vi "MTDC_Prototype.vi"() -> ()   [LabVIEW 2025]
uses:
  STM-Auto-Project/QMH CTLS/Scan_Params (QMH).ctl
  <instrlib>/SMS LabVIEW Drivers/Source Code/Public/PSU Status.ctl
  <instrlib>/SMS LabVIEW Drivers/Source Code/Cryogenic Ltd SMSXXX.lvlib
  Downloads/OneDrive_2025-09-03/Instrument Controls/Temp Cntrl.ctl
  STM-Auto-Project/QMH CTLS/Sweeper.ctl
  Magnetic Drift Correction/XY_Coords(Final).ctl
panel:
  out "Polled Temps (K)":dbl[](array[numeric])
  in  "Serial Configuration":T1={"Baud Rate"=57600, "Parity"=1, "Data Bits"=7, "Stop Bits"=10, "Flow Control"=0}
  out "Translation (m)":T2
  out "Final coordinates (m)":cluster{"Xc":sgl, "Yc":sgl} {"Yc" format="%.4p"; "Xc" format="%.4p"}
  out "Initial coordinates (m)":cluster{"Xc":sgl, "Yc":sgl} {"Yc" format="%.4p"; "Xc" format="%.4p"}
  in  "Field and Temp Range":T3={"VISA (Magnet)"="COM4", "Fields(T)"=[], "Temps(K)"=[], "VISA (Temp) "="COM1", "Port number (3364)"=3364}
  in  "Lead- Mode Ramp Rate (A/s)":dbl=0.02
  out "Errors":errorcluster[](array[cluster])
  out "Output (T)":dbl
  in  "P-Mode Ramp Rate (A/s)":dbl
  out "MID Setpoint (T)":dbl
  out "Current Index":i32
  in  "stop":bool
  in  "Start":bool
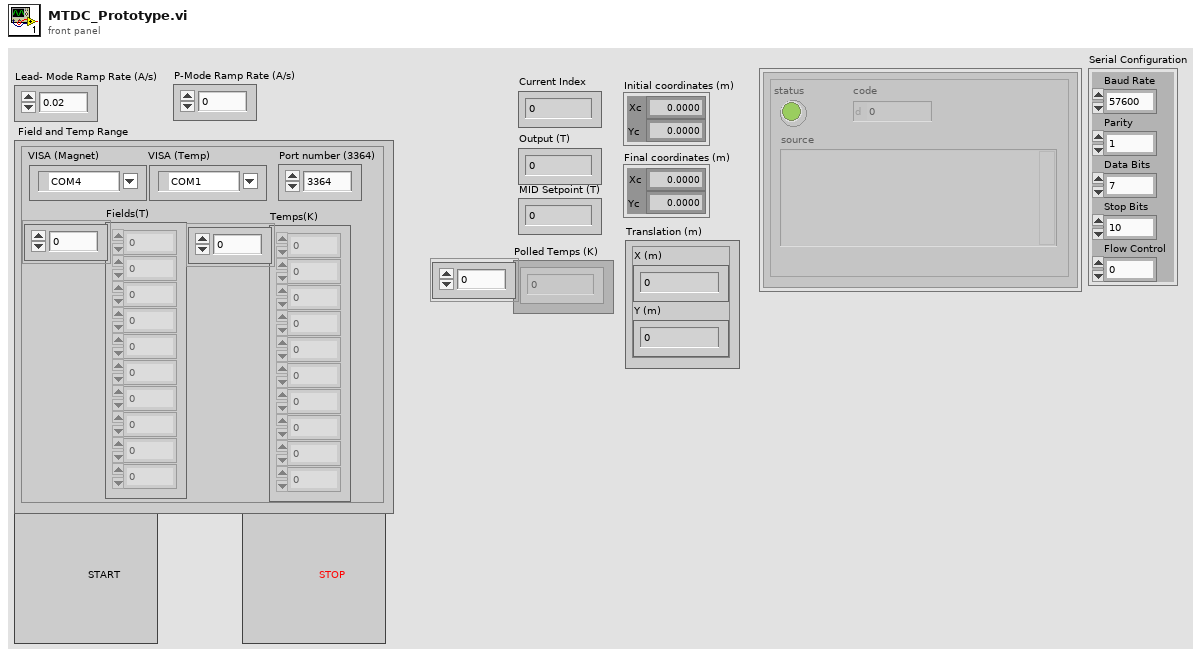
[diagram p1: front panel]
types:
  T1 = cluster{"Baud Rate":u32, "Parity":u16, "Data Bits":u16, "Stop Bits":u16, "Flow Control":u16}
  T2 = typedef "XY_Coords(Final).ctl" = cluster{"X (m)":dbl, "Y (m)":dbl}
  T3 = cluster{"VISA (Magnet)":refnum<visa-resource-name>, "Fields(T)":dbl[], "Temps(K)":dbl[], "VISA (Temp) ":refnum<visa-resource-name>, "Port number (3364)":u32}
  T4 = enum16{"NO CHANGE", "SET TEMP & FIELD", "SWEEP IDLE", "NEXT TEMP & FIELD", "SWEEP DONE"}
  T5 = enum16{"1. BIAS", "2. INIT_SCAN", "3. SCAN_IDLE", "4. INTER_SCAN", "5. NEW_COORDS_&_FRAME", "6. FINAL_SCAN", "7. POLL BIAS ", "8. STOP"}
  T6 = typedef "Sweeper.ctl" = cluster{"Temps(K)":dbl[], "Fields(T)":dbl[], "Sweep States":enum16{"NO CHANGE", "SET TEMP & FIELD", "SWEEP IDLE", "NEXT TEMP & FIELD", "SWEEP DONE"}}
  T7 = enum16{"1. INIT TEMP", "2. TC ON", "3. POLL_TEMPS", "4. TEMP_STAB", "5. TC IDLE", "6. APPLY NEXT TEMP", "7. TC OFF (Reset)"}
  T8 = typedef "Temp Cntrl.ctl" = cluster{"Range (0:Off)":u16, "Manual Output (0.00 %)":dbl, "Rate (D) (0.0 %)":dbl, "Reset (I) (20.0)":dbl, "Gain (P) (50.0)":dbl, "Power Up Enable (F: Disable)":bool, "Max User Current (2.000)":dbl, "Heater Resistance (1:25 Ohms)":u16, "Max Current (0:User Specified)":u16, "Heater Out Display (1:Current)":u16, "Mode (0:Off)":u16, "Input (0:None)":u16, "Target Temp (K)":dbl, "Serial Configuration":cluster{"Baud Rate":u32, "Parity":u16, "Data Bits":u16, "Stop Bits":u16, "Flow Control":u16}, "VISA resource name":refnum<visa-resource-name>, "Configure Control Parameters (0: Configure)":u16, "Enable Setpoint (F:Disable)":bool, "Input (0:A)":u16, "Data Source (0:Kelvin)":u16, "Output's Control Loop (1:1)":u16, "STND DEV Threshold ":dbl, "Mean Tolerance ":dbl, "Current State":enum16{"1. INIT TEMP", "2. TC ON", "3. POLL_TEMPS", "4. TEMP_STAB", "5. TC IDLE", "6. APPLY NEXT TEMP", "7. TC OFF (Reset)"}}
  T9 = enum16{"1. INIT MAG", "2. MAG ON", "3. MAG_STAB", "4. MAG IDLE", "5. PREP NEXT FIELD", "6. APPLY NEXT FIELD", "7. PREP OFF", "8. MAG OFF (Reset)"}
  T10 = typedef "PSU Status.ctl" = cluster{"Ramp Target":enum16{"ZERO", "MID", "MAX"}, "Pause":bool, "Switch Heater":bool, "Persistent Field":dbl, "Persistent Current":dbl, "Tesla":bool, "Output (T)":dbl, "Output (A)":dbl, "X Trip":enum16{"DISABLED", "ENABLED", "ACTIVE"}, "Ramp Rate (A/s)":dbl, "V Limit (V)":dbl, "Heater Voltage":dbl, "MAX Setpoint (A)":dbl, "MAX Setpoint (T)":dbl, "MID Setpoint (A)":dbl, "MID Setpoint (T)":dbl, "Lock":bool, "Field Constant":dbl, "Remote":bool, "Direction":enum16{"POSITIVE", "NEGATIVE", "OPEN", "UNIPOLAR"}, "Helium Level":u16, "Quench !":bool, "Voltage":dbl, "V Limit !":bool, "Ramping":bool, "At Target":bool, "Trip Field":dbl, "Trip Current":dbl, "Current State":enum16{"1. INIT MAG", "2. MAG ON", "3. MAG_STAB", "4. MAG IDLE", "5. PREP NEXT FIELD", "6. APPLY NEXT FIELD", "7. PREP OFF", "8. MAG OFF (Reset)"}, "MAG Reference":refnum<visa-resource-name>}
  T11 = typedef "Scan_Params (QMH).ctl" = cluster{"Setpoint (I)":dbl[], "Bias (V)":dbl[], "Number of scans":u8, "Port number (3364)":u32, "Avoid zero threshold (V)":dbl, "Current State":enum16{"1. BIAS", "2. INIT_SCAN", "3. SCAN_IDLE", "4. INTER_SCAN", "5. NEW_COORDS_&_FRAME", "6. FINAL_SCAN", "7. POLL BIAS ", "8. STOP"}}
  T12 = enum16{"RAMP TO ZERO", "RAMP TO MID", "RAMP TO MAX"}
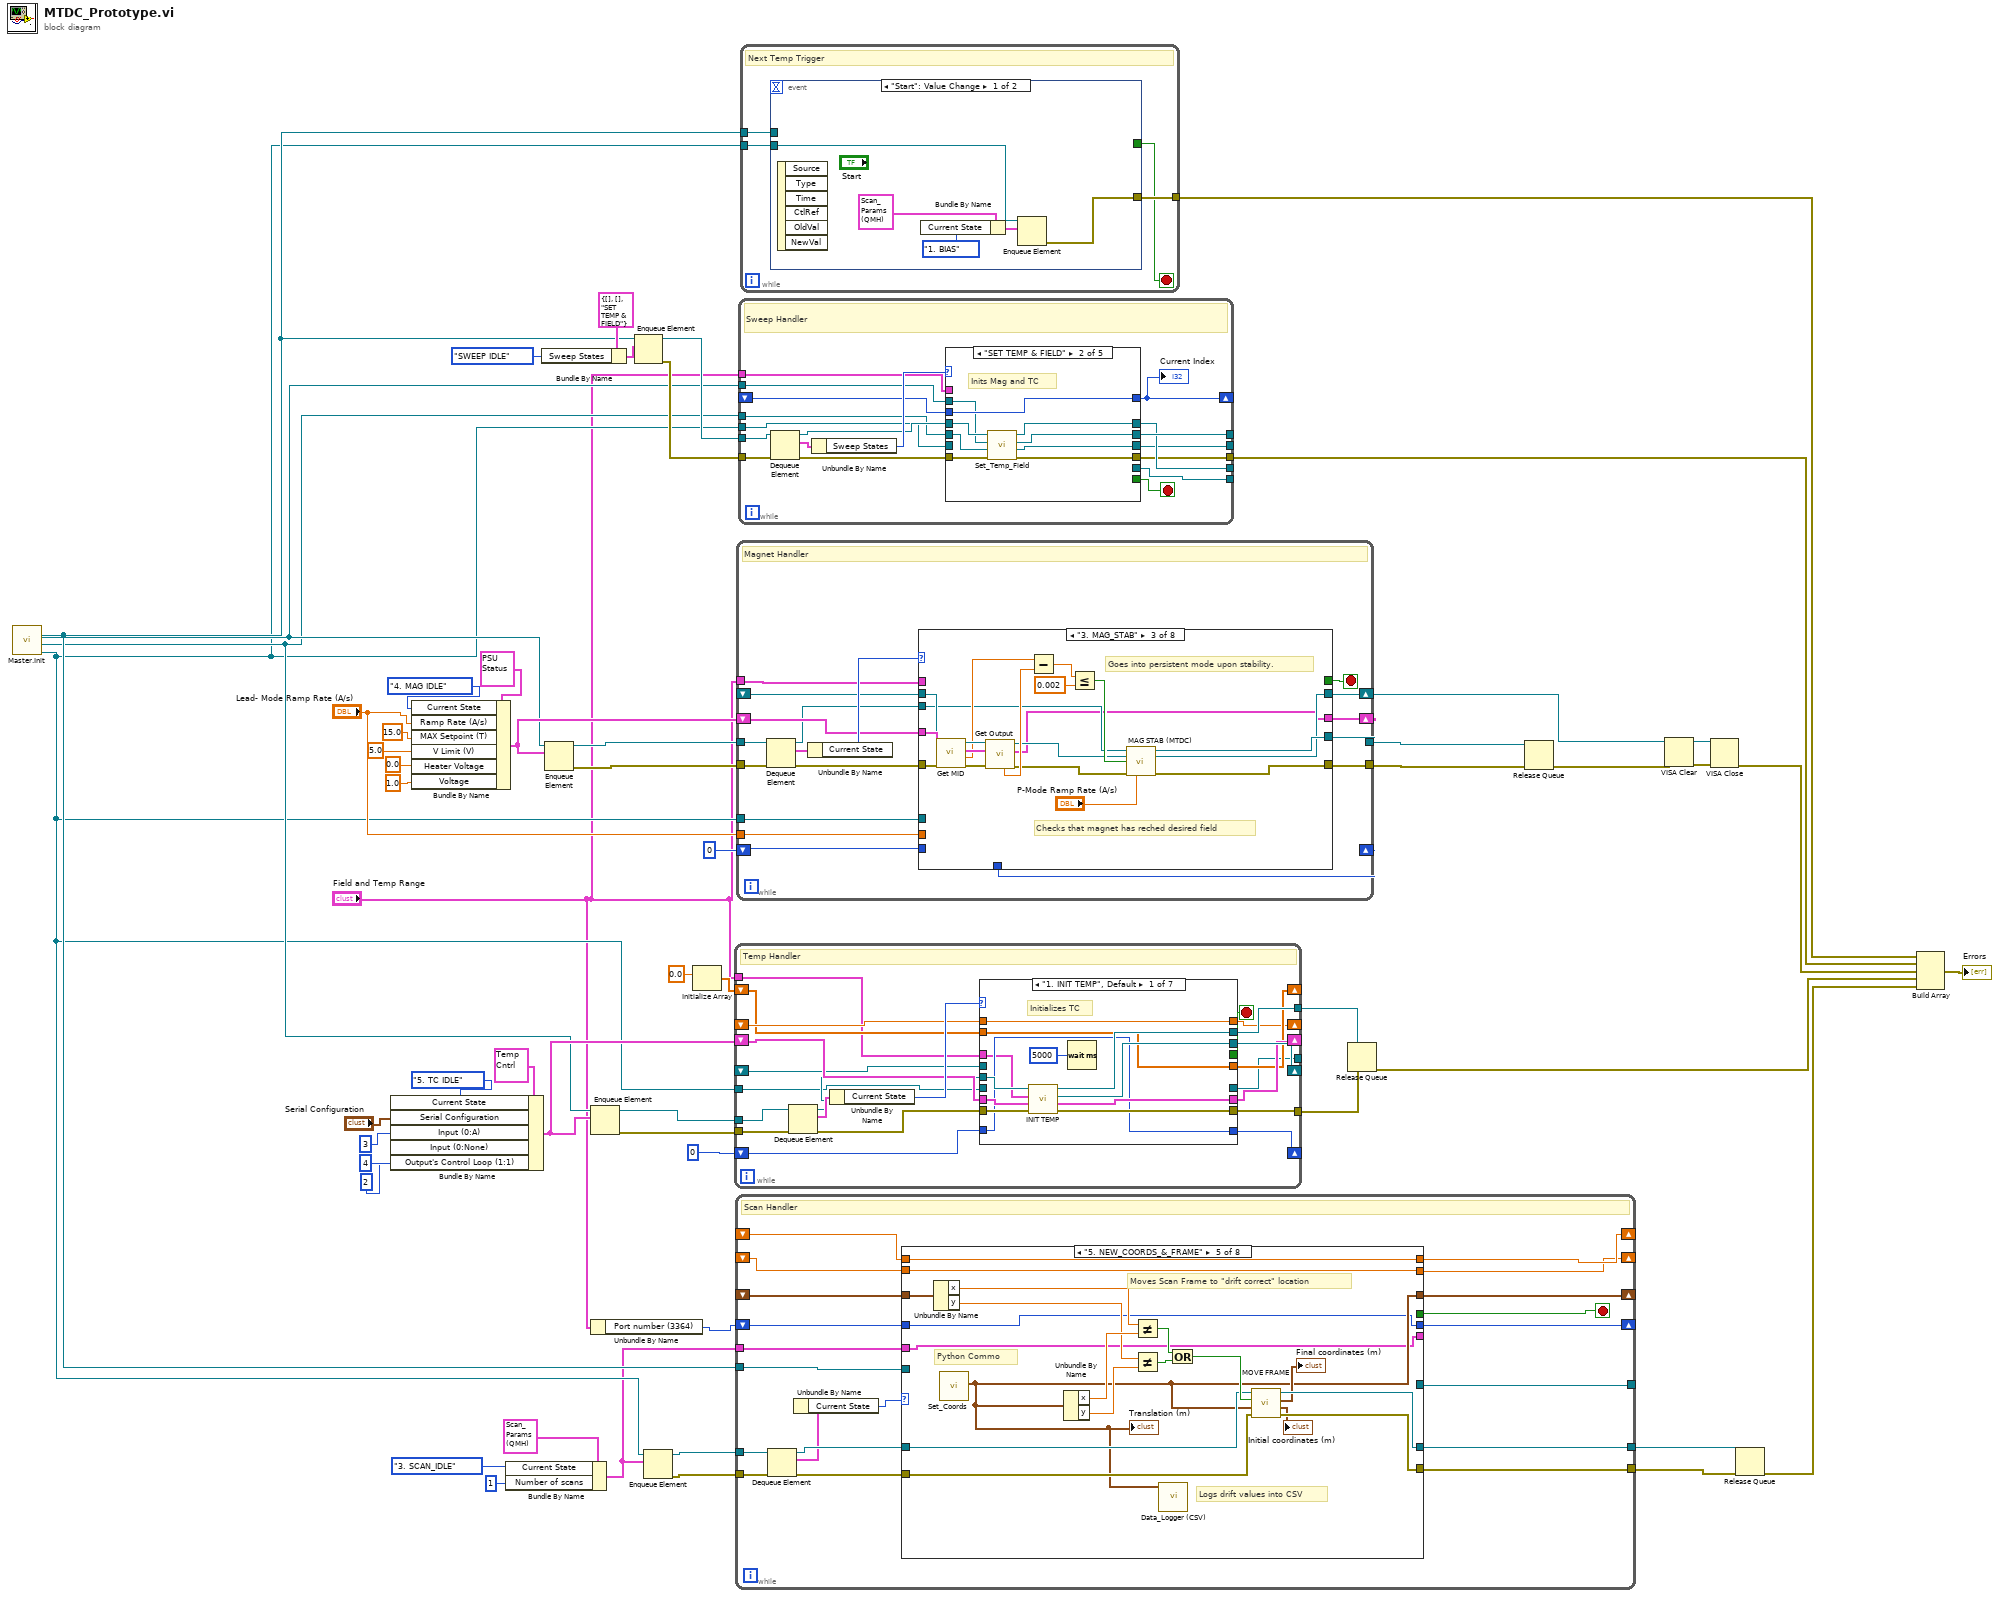
[diagram p0: block diagram]
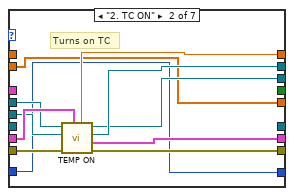
[diagram p2: hidden frame]
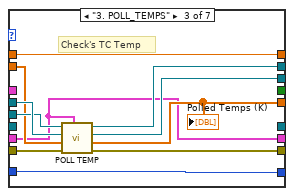
[diagram p3: hidden frame]
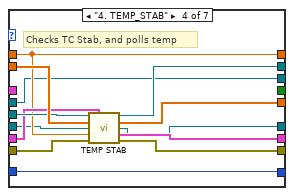
[diagram p4: hidden frame]
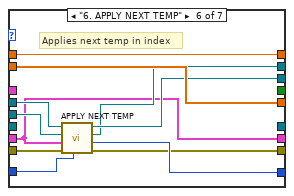
[diagram p6: hidden frame]
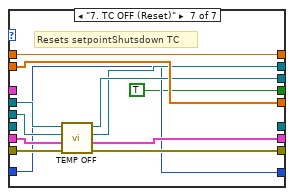
[diagram p7: hidden frame]
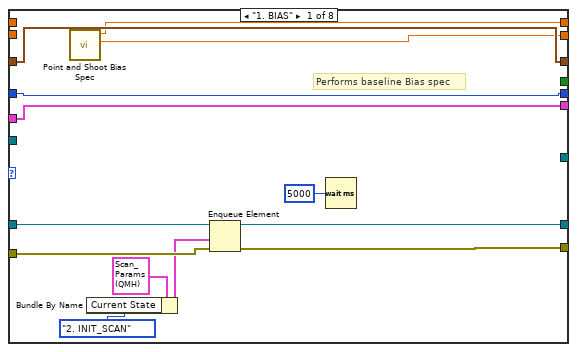
[diagram p8: hidden frame]
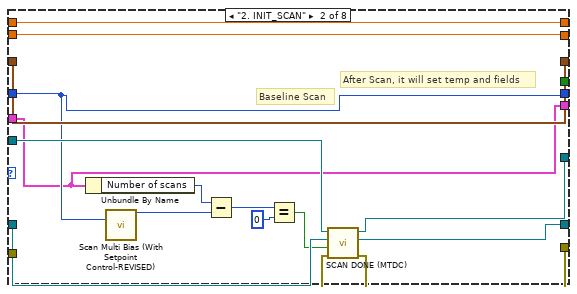
[diagram p9: hidden frame]
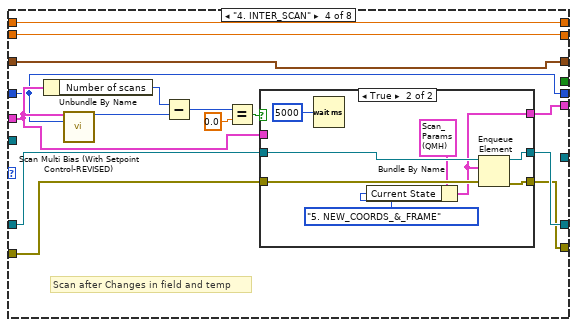
[diagram p11: hidden frame]
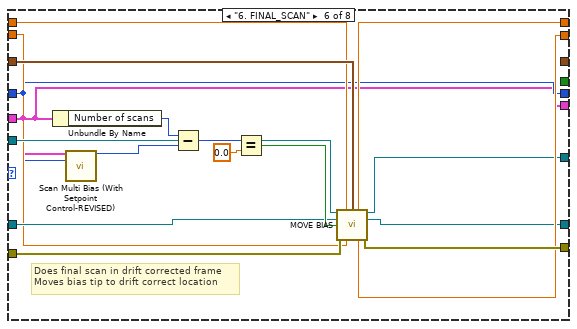
[diagram p13: hidden frame]
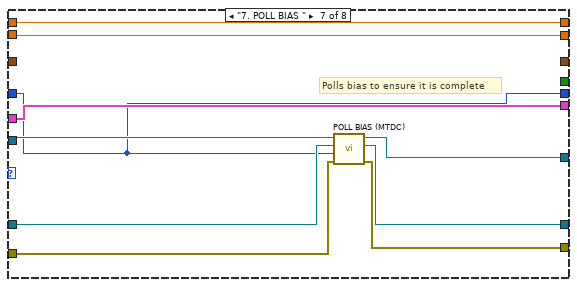
[diagram p14: hidden frame]
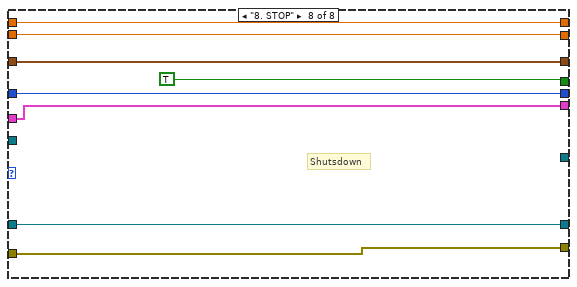
[diagram p15: hidden frame]
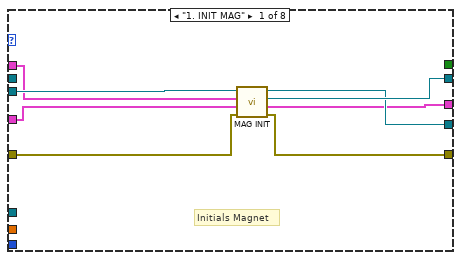
[diagram p16: hidden frame]
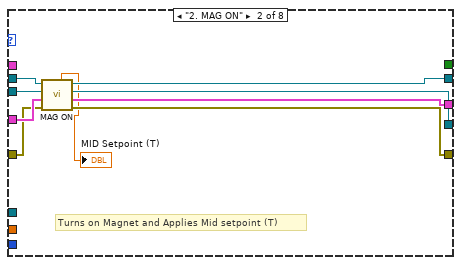
[diagram p17: hidden frame]
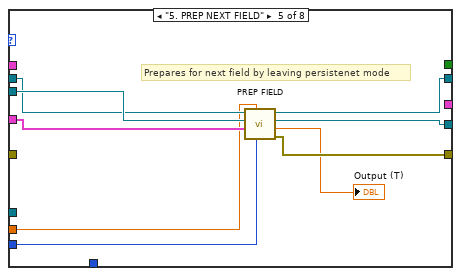
[diagram p19: hidden frame]
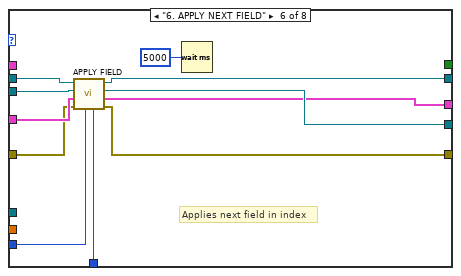
[diagram p20: hidden frame]
diagram:
  n1 = call "Master.Init.vi"() -> ("ScanQ"=w5:refnum<queue>, "TempQ"=w8:refnum<queue>, "MagQ"=w13:refnum<queue>, "SweepQ"=w14:refnum<queue>)  [unwired: 8 in]
  n2 = Bundle By Name(cluster=T8 {"Range (0:Off)"=0, "Manual Output (0.00 %)"=0.0, "Rate (D) (0.0 %)"=0.0, "Reset (I) (20.0)"=20.0, "Gain (P) (50.0)"=50.0, "Power Up Enable (F: Disable)"=FALSE, "Max User Current (2.000)"=2.0, "Heater Resistance (1:25 Ohms)"=1, "Max Current (0:User Specified)"=0, "Heater Out Display (1:Current)"=1, "Mode (0:Off)"=1, "Input (0:None)"=4, "Target Temp (K)"=5.0, "Serial Configuration"={"Baud Rate"=57600, "Parity"=1, "Data Bits"=7, "Stop Bits"=10, "Flow Control"=0}, "VISA resource name"="", "Configure Control Parameters (0: Configure)"=0, "Enable Setpoint (F:Disable)"=FALSE, "Input (0:A)"=3, "Data Source (0:Kelvin)"=0, "Output's Control Loop (1:1)"=2, "STND DEV Threshold "=0.1, "Mean Tolerance "=0.02, "Current State"=enum."1. INIT TEMP"} ("element"), "Current State"=T7."5. TC IDLE", "Serial Configuration"="Serial Configuration", "Input (0:A)"=u16 3, "Input (0:None)"=u16 4, "Output's Control Loop (1:1)"=u16 2) -> (w23:T8)
  n3 = Bundle By Name(cluster=T10 {"Ramp Target"=enum."ZERO", "Pause"=FALSE, "Switch Heater"=FALSE, "Persistent Field"=0.0, "Persistent Current"=0.0, "Tesla"=FALSE, "Output (T)"=0.0, "Output (A)"=0.0, "X Trip"=enum."DISABLED", "Ramp Rate (A/s)"=0.0, "V Limit (V)"=0.0, "Heater Voltage"=0.0, "MAX Setpoint (A)"=0.0, "MAX Setpoint (T)"=0.0, "MID Setpoint (A)"=0.0, "MID Setpoint (T)"=0.0, "Lock"=FALSE, "Field Constant"=0.0, "Remote"=FALSE, "Direction"=enum."POSITIVE", "Helium Level"=0, "Quench !"=FALSE, "Voltage"=0.0, "V Limit !"=FALSE, "Ramping"=FALSE, "At Target"=FALSE, "Trip Field"=0.0, "Trip Current"=0.0, "Current State"=enum."1. INIT MAG", "MAG Reference"="COM4"} ("PSU Status In"), "Current State"=T9."4. MAG IDLE", "Ramp Rate (A/s)"="Lead- Mode Ramp Rate (A/s)", "MAX Setpoint (T)"=15.0, "V Limit (V)"=5.0, "Heater Voltage"=0.0, "Voltage"=1.0) -> (w47:T10)
  n4 = Bundle By Name(cluster=T11 {"Setpoint (I)"=[], "Bias (V)"=[], "Number of scans"=1, "Port number (3364)"=3364, "Avoid zero threshold (V)"=0.004999999888241291, "Current State"=enum."1. BIAS"} ("element"), "Current State"=T5."3. SCAN_IDLE", "Number of scans"=u8 1) -> (w2:T11)
  n5 = Bundle By Name(cluster=T6 {"Temps(K)"=[], "Fields(T)"=[], "Sweep States"=enum."SET TEMP & FIELD"} ("Temp and Field Range"), "Sweep States"=T4."SWEEP IDLE") -> (w12:T6)
  n6 = Enqueue Element(queue=w13, element=w47) -> (queue out=w50:refnum<queue>, error out=w49:errorcluster)  [unwired: 2 in, 1 out]
  n7 = Enqueue Element(queue=w8, element=w23) -> (queue out=w27:refnum<queue>, error out=w7:errorcluster)  [unwired: 2 in, 1 out]
  n8 = Unbundle By Name("Field and Temp Range") -> ("Port number (3364)"=w3:u32)
  n9 = Enqueue Element(queue=w14, element=w12) -> (queue out=w52:refnum<queue>, error out=w51:errorcluster)  [unwired: 2 in, 1 out]
  n10 = Enqueue Element(queue=w5, element=w2) -> (queue out=w38:refnum<queue>, error out=w37:errorcluster)  [unwired: 2 in, 1 out]
  n11 = Initialize Array(0.0 ("element")) -> (w20:dbl[])  [unwired: 1 in]
  n12 = while {
    tunnel: w27 -> [w78]
    tunnel: w7 -> [w77]
    shift-right: [w68] -> _
    shift-left: w23 -> [w74]
    shift-right: [w72] -> _
    shift-left: _ -> [w67]
    tunnel: [w71] -> w16
    tunnel: [w69] -> w17
    shift-right: [w63] -> _
    shift-left: _ -> [w66]
    shift-right: [w64] -> _
    shift-left: w20 -> [w65]
    tunnel: [w62] -> _
    shift-right: [w60] -> _
    shift-left: 0 -> [w61]
    tunnel: w5 -> [w58]
    tunnel: "Field and Temp Range" -> [w57]
    stop <- w59 stop-if-true
    # "Temp Handler"
    n13 = Dequeue Element(queue=w78, error in (no error)=w77) -> (queue out=w70:refnum<queue>, element=w76:T8, error out=w73:errorcluster)  [unwired: 1 in, 1 out]
    n14 = Unbundle By Name(w76) -> ("Current State"=w75:T7)
    n15 = case shown="\"1. INIT TEMP\", Default" w75 {
      tunnel: w74 -> [w90 w101 w102 w123 w127 w133 w150]
      tunnel: w73 -> [w89 w95 w111 w122 w128 w138 w153]
      tunnel: [w88 w94 w110 w114 w129 w137 w152] -> w72
      tunnel: [w85 w98 w107 w120 w128 w134 w149] -> w71
      tunnel: w70 -> [w87 w100 w109 w124 w130 w136 w151]
      tunnel: [w86 w99 w108 w121 w130 w135 w148] -> w69
      tunnel: [w83 w97 w102 w117 w127 w133 w147] -> w68
      tunnel: w67 -> [_ w96 w112 w114 w129 w139 w154]
      tunnel: [w81 w93 w104 w118 w131 w142 w145] -> w63
      tunnel: w66 -> [w81 _ w104 w118 w131 w142 w145]
      tunnel: w65 -> [w82 w92 w106 w125 w132 w143 w155]
      tunnel: [w82 w92 w105 w119 w132 w143 w155] -> w64
      tunnel: [_ _ _ w116 _ _ _] -> w62
      tunnel: w61 -> [w80 w91 w103 w115 w126 w141 w146]
      tunnel: [w80 w91 w103 w115 w126 w140 w146] -> w60
      tunnel: [_ _ _ _ _ _ TRUE] -> w59
      tunnel: w58 -> [_ _ _ w113 _ _ _]
      tunnel: w57 -> [w79 _ _ _ _ _ _]
      frame "1. INIT TEMP", Default {
        # "Initializes TC"
        n16 = call "INIT TEMP.vi"("error in (no error)"=w89, "element"=w90, "Field and Temp Range"=w79, "Queue in"=w87) -> ("error out"=w85:errorcluster, "output cluster"=w83:T8, "VISA resource name out"=w88:refnum<visa-resource-name>, "Queue out"=w86:refnum<queue>)  [unwired: 4 in]
        n17 = Wait (ms)(milliseconds to wait=u32 5000) -> ()  [unwired: 1 out]
      }
      frame "2. TC ON" {
        # "Turns on TC"
        n18 = call "TEMP ON.vi"("element in"=w101, "error in (no error)"=w95, "TempQ in"=w100, "VISA Refnum in"=w96) -> ("error out"=w98:errorcluster, "element out"=w97:T8, "TempQ out"=w99:refnum<queue>, "VISA Refnum out"=w94:refnum<visa-resource-name>, "Setpoint"=w93:dbl)  [unwired: 3 in]
      }
      frame "3. POLL_TEMPS" {
        # "Check's TC Temp"
        n19 = call "POLL TEMP.vi"("element"=w102, "error in (no error)"=w111, "Array in"=w106, "VISA resource name in"=w112, "Queue in"=w109) -> ("error out"=w107:errorcluster, "Array"=w105:dbl[], "VISA resource name out"=w110:refnum<visa-resource-name>, "Queue out"=w108:refnum<queue>)  [unwired: 3 in]
        "Polled Temps (K)" <- w105
      }
      frame "4. TEMP_STAB" {
        # "Checks TC Stab, and polls temp"
        n20 = call "TEMP STAB.vi"("Queue in"=w124, "element in"=w123, "Array in"=w125, "ScanQ In"=w113, "Setpoint"=w118, "error in (no error)"=w122) -> ("Queue out"=w121:refnum<queue>, "Array out"=w119:dbl[], "ScanQ"=w116:refnum<queue>, "element out"=w117:T8, "error out"=w120:errorcluster)  [unwired: 5 in]
      }
      frame "5. TC IDLE" {
      }
      frame "6. APPLY NEXT TEMP" {
        # "Applies next temp in index"
        n21 = call "APPLY NEXT TEMP.vi"("Numeric in"=w141, "error in (no error)"=w138, "element in"=w133, "TempQ in"=w136, "VISA Refnum in"=w139) -> ("error out"=w134:errorcluster, "Numeric out"=w140:i32, "TempQ out"=w135:refnum<queue>, "VISA Refnum out"=w137:refnum<visa-resource-name>)  [unwired: 3 in]
      }
      frame "7. TC OFF (Reset)" {
        # "Resets setpointShutsdown TC"
        n22 = call "TEMP OFF.vi"("error in (no error)"=w153, "element in"=w150, "TempQ in"=w151, "VISA Refnum in"=w154) -> ("error out"=w149:errorcluster, "element out"=w147:T8, "TempQ out"=w148:refnum<queue>, "VISA Refnum out"=w152:refnum<visa-resource-name>)  [unwired: 4 in]
      }
    }
  }
  n23 = while {
    tunnel: w37 -> [w168]
    shift-right: [w156] -> _
    shift-left: w3 -> [w175]
    tunnel: [w174] -> w36
    shift-right: [w172] -> _
    shift-left: _ -> [w171]
    tunnel: [w169] -> w35
    tunnel: [w166] -> _
    tunnel: w38 -> [w165]
    tunnel: w14 -> [w164]
    shift-right: [w163] -> _
    shift-left: _ -> [w161]
    shift-right: [w162] -> _
    shift-left: _ -> [w160]
    tunnel: w2 -> [w157]
    stop <- w170 stop-if-true
    # "Scan Handler"
    n24 = Dequeue Element(queue=w165, error in (no error)=w168) -> (queue out=w173:refnum<queue>, element=w159:T11, error out=w167:errorcluster)  [unwired: 1 in, 1 out]
    n25 = Unbundle By Name(w159) -> ("Current State"=w158:T5)
    n26 = case shown="\"5. NEW_COORDS_&_FRAME\"" w158 {
      tunnel: w175 -> [w177 w190 w206 w211 w237 w257 w274 w285]
      tunnel: [w187 w198 w209 w220 w247 w259 w280 w290] -> w174
      tunnel: w167 -> [w183 w196 _ w216 w244 w267 w278 w289]
      tunnel: w173 -> [w188 w199 w209 w221 w248 w265 w282 w290]
      tunnel: [w176 w189 w205 w219 w238 w256 w275 w284] -> _
      tunnel: [w186 w201 w210 w218 w241 _ _ w288] -> w172
      tunnel: w171 -> [w186 w201 w210 w218 w246 w269 _ w288]
      tunnel: [_ _ _ _ _ _ _ TRUE] -> w170
      tunnel: [w184 w195 _ w217 w245 w268 w279 w289] -> w169
      tunnel: [_ w197 _ _ _ w260 w281 _] -> w166
      tunnel: w164 -> [_ w200 _ _ _ w266 w283 _]
      tunnel: [w180 w193 w208 w215 w240 w262 w277 w286] -> w163
      tunnel: [w179 w192 w207 w214 w239 w261 w276 w287] -> w162
      tunnel: w161 -> [_ w193 w208 w215 w240 w264 w277 w286]
      tunnel: w160 -> [_ w192 w207 w214 w239 w263 w276 w287]
      tunnel: w157 -> [w176 w189 w205 w212 w238 w256 w275 w284]
      tunnel: [w177 w190 w206 w211 w237 w257 w274 w285] -> w156
      frame "1. BIAS" {
        # "Performs baseline Bias spec"
        n27 = call "Point and Shoot Bias Spec.vi"() -> ("Initial Y (m)"=w179:dbl, "Inital X (m)"=w180:dbl)  [unwired: 10 in]
        n28 = Bundle By Name(cluster=T11 {"Setpoint (I)"=[], "Bias (V)"=[], "Number of scans"=1, "Port number (3364)"=3364, "Avoid zero threshold (V)"=0.004999999888241291, "Current State"=enum."1. BIAS"} ("element"), "Current State"=T5."2. INIT_SCAN") -> (w181:T11)
        n29 = Enqueue Element(queue=w188, element=w181, error in (no error)=w183) -> (queue out=w187:refnum<queue>, error out=w184:errorcluster)  [unwired: 1 in, 1 out]
        n30 = Wait (ms)(milliseconds to wait=u32 5000) -> ()  [unwired: 1 out]
      }
      frame "2. INIT_SCAN" {
        # "Baseline Scan"
        # "After Scan, it will set temp and fields"
        n31 = Unbundle By Name(w189) -> ("Number of scans"=w191:u8)
        n32 = call "Scan Multi Bias (With Setpoint Control-REVISED).vi"("Port number (3364)"=w190) -> ("Scan"=w202:u8)  [unwired: 13 in, 1 out]
        n33 = Subtract(x=w191, y=w202) -> (x-y=w204:u8)
        n34 = Equal?(x=w204, y=u8 0) -> (x = y?=w194:bool)
        n35 = call "SCAN DONE (MTDC).vi"("error in (no error)"=w196, "Boolean"=w194, "ScanQ in"=w199, "SweepQ"=w200) -> ("error out"=w195:errorcluster, "ScanQ out"=w198:refnum<queue>, "SweepQ out"=w197:refnum<queue>)  [unwired: 5 in]
      }
      frame "3. SCAN_IDLE" {
      }
      frame "4. INTER_SCAN" {
        # "Scan after Changes in field and temp"
        n36 = Unbundle By Name(w212) -> ("Number of scans"=w213:u8)
        n37 = call "Scan Multi Bias (With Setpoint Control-REVISED).vi"("Scan Parameters"=w212, "Port number (3364)"=w211) -> ("Scan"=w222:u8)  [unwired: 12 in, 1 out]
        n38 = Subtract(x=w213, y=w222) -> (x-y=w224:u8)
        n39 = Equal?(x=w224, y=0.0) -> (x = y?=w223:bool)
        n40 = case shown="True" w223 {
          tunnel: w221 -> [w228 w235]
          tunnel: [w228 w234] -> w220
          tunnel: [w226 w229] -> w219
          tunnel: [w227 w233] -> w217
          tunnel: w216 -> [w227 w232]
          tunnel: w212 -> [w226 _]
          frame False {
          }
          frame True {
            n41 = Wait (ms)(milliseconds to wait=u32 5000) -> ()  [unwired: 1 out]
            n42 = Bundle By Name(cluster=T11 {"Setpoint (I)"=[], "Bias (V)"=[], "Number of scans"=1, "Port number (3364)"=3364, "Avoid zero threshold (V)"=0.004999999888241291, "Current State"=enum."2. INIT_SCAN"} ("element"), "Current State"=T5."5. NEW_COORDS_&_FRAME") -> (w229:T11)
            n43 = Enqueue Element(queue=w235, element=w229, error in (no error)=w232) -> (queue out=w234:refnum<queue>, error out=w233:errorcluster)  [unwired: 1 in, 1 out]
          }
        }
      }
      frame "5. NEW_COORDS_&_FRAME" {
        # "Python Commo"
        # "Logs drift values into CSV"
        # "Moves Scan Frame to \"drift correct\" location"
        n44 = Unbundle By Name(w246) -> ("x"=w250:dbl, "y"=w249:dbl)
        n45 = call "Set_Coords.vi"() -> ("return value"=w241:cluster{"x":dbl, "y":dbl})  [unwired: 10 in, 1 out]
        "Translation (m)" <- w241
        n46 = Unbundle By Name(w241) -> ("x"=w253:dbl, "y"=w252:dbl)
        n47 = Not Equal?(x=w250, y=w253) -> (x != y?=w255:bool)
        n48 = Not Equal?(x=w249, y=w252) -> (x != y?=w254:bool)
        n49 = call "Data_Logger (CSV).vi"("Translation (m)"=w241) -> ()  [unwired: 11 in]
        n50 = Or(x=w255, y=w254) -> (x .or. y?=w251:bool)
        n51 = call "MOVE FRAME.vi"("error in (no error)"=w244, "return value"=w241, "Boolean"=w251, "Queue in"=w248) -> ("error out"=w245:errorcluster, "Initial coordinates (m)"=→"Initial coordinates (m)":cluster{"Xc":sgl, "Yc":sgl}, "Final coordinates (m)"=→"Final coordinates (m)":cluster{"Xc":sgl, "Yc":sgl}, "Queue out"=w247:refnum<queue>)  [unwired: 4 in]
      }
      frame "6. FINAL_SCAN" {
        # "Does final scan in drift corrected frame\nMoves bias tip to drift correct location"
        n52 = Unbundle By Name(w256) -> ("Number of scans"=w258:u8)
        n53 = call "Scan Multi Bias (With Setpoint Control-REVISED).vi"("Scan Parameters"=w256, "Port number (3364)"=w257) -> ("Scan"=w271:u8)  [unwired: 12 in, 1 out]
        n54 = Subtract(x=w258, y=w271) -> (x-y=w272:u8)
        n55 = Equal?(x=w272, y=0.0) -> (x = y?=w270:bool)
        n56 = call "MOVE BIAS.vi"("SweepQ in"=w266, "x"=w264, "return value"=w269, "ScanQ in"=w265, "Boolean"=w270, "error in (no error)"=w267, "y"=w263) -> ("X (m)"=w262:sgl, "SweepQ out"=w260:refnum<queue>, "ScanQ out"=w259:refnum<queue>, "Y (m)"=w261:sgl, "error out"=w268:errorcluster)  [unwired: 4 in]
      }
      frame "7. POLL BIAS " {
        # "Polls bias to ensure it is complete"
        n57 = call "POLL BIAS (MTDC).vi"("error in (no error)"=w278, "Port number (3364)"=w274, "ScanQ in"=w282, "SweepQ in"=w283) -> ("error out"=w279:errorcluster, "ScanQ out"=w280:refnum<queue>, "SweepQ out"=w281:refnum<queue>)  [unwired: 5 in]
      }
      frame "8. STOP" {
        # "Shutsdown"
      }
    }
  }
  n58 = while {
    tunnel: w50 -> [w308]
    tunnel: [w304] -> w55
    shift-right: [w303] -> _
    shift-left: w47 -> [w306]
    shift-right: [w302] -> w32
    shift-left: _ -> [w301]
    tunnel: [w300] -> w56
    tunnel: w49 -> [w299]
    tunnel: "Field and Temp Range" -> [w298]
    shift-right: [w293] -> _
    shift-left: 0 -> [w297]
    tunnel: "Lead- Mode Ramp Rate (A/s)" -> [w295]
    tunnel: w5 -> [w294]
    stop <- w292 stop-if-true
    # "Magnet Handler"
    n59 = Dequeue Element(queue=w308, error in (no error)=w299) -> (queue out=w296:refnum<queue>, element=w309:T10, error out=w305:errorcluster)  [unwired: 1 in, 1 out]
    n60 = Unbundle By Name(w309) -> ("Current State"=w307:T9)
    n61 = case "MAG STATE MACHINE" shown="\"3. MAG_STAB\"" w307 {
      tunnel: w306 -> [w313 w326 w344 w349 w355 w365 w390 w405]
      tunnel: w305 -> [w311 w324 w345 w348 _ w364 w389 w406]
      tunnel: [w316 w321 w328 w348 w352 w368 w370 w393] -> w304
      tunnel: [w314 w322 w327 w349 _ w361 w371 w396] -> w303
      tunnel: [w317 w323 w331 w347 w351 w362 w373 w397] -> w302
      tunnel: w301 -> [_ w325 w343 w347 w354 w366 w391 w407]
      tunnel: [w315 w320 w332 w346 w357 w369 w372 w395] -> w300
      tunnel: w298 -> [w310 _ _ _ _ _ _ _]
      tunnel: w297 -> [_ _ _ _ w358 w363 _ _]
      tunnel: w296 -> [w312 w319 w333 w346 w356 w360 w381 w400]
      tunnel: w295 -> [_ _ _ _ w353 _ _ _]
      tunnel: w294 -> [_ _ _ _ _ _ _ _]
      tunnel: [_ _ _ _ _ w359 _ _] -> w293
      tunnel: [_ _ _ _ _ _ _ w394] -> w292
      frame "1. INIT MAG" {
        # "Initials Magnet"
        n62 = call "MAG INIT.vi"("error in (no error)"=w311, "PSU Status In"=w313, "Field and Temp Range"=w310, "Queue in"=w312) -> ("error out"=w316:errorcluster, "PSU Status Out"=w314:T10, "VISA Resource Name Out"=w317:refnum<visa-resource-name>, "Queue out"=w315:refnum<queue>)  [unwired: 4 in]
      }
      frame "2. MAG ON" {
        # "Turns on Magnet and Applies Mid setpoint (T)"
        n63 = call "MAG ON.vi"("error in (no error)"=w324, "PSU Status In"=w326, "MagQ in"=w319, "VISA Refnum in"=w325) -> ("error out"=w321:errorcluster, "PSU Status Out"=w322:T10, "MagQ out"=w320:refnum<queue>, "VISA Refnum out"=w323:refnum<visa-resource-name>, "MID Setpoint (T)"=→"MID Setpoint (T)":dbl)  [unwired: 3 in]
      }
      frame "3. MAG_STAB" {
        # "Checks that magnet has reched desired field"
        # "Goes into persistent mode upon stability."
        n64 = call <instrlib>:"Get MID.vi"("Error in (no error)"=w345, "PSU Status In"=w344, "VISA Resource Name In"=w343) -> ("Error out"=w342:errorcluster, "MID Setpoint (T)"=w338:dbl, "PSU Status Out"=w341:T10, "VISA Resource Name Out"=w340:refnum<visa-resource-name>)  [unwired: 3 in, 2 out]
        n65 = call <instrlib>:"Get Output.vi"("Error in (no error)"=w342, "PSU Status In"=w341, "VISA Resource Name In"=w340) -> ("Error out"=w329:errorcluster, "PSU Status Out"=w327:T10, "VISA Resource Name Out"=w330:refnum<visa-resource-name>, "Output (T)"=w336:dbl)  [unwired: 3 in, 2 out]
        n66 = Subtract(x=w338, y=w336) -> (x-y=w337:dbl)
        n67 = Less Or Equal?(x=w337, y=0.002) -> (x <= y?=w335:bool)
        n68 = call "MAG STAB (MTDC).vi"("MagQ"=w333, "VISA In"=w330, "Boolean"=w335, "Error out"=w329, "P-Mode Ramp Rate (A/s)"="P-Mode Ramp Rate (A/s)") -> ("MagQ"=w332:refnum<queue>, "VISA Out"=w331:refnum<visa-resource-name>, "error out"=w328:errorcluster)  [unwired: 8 in]
      }
      frame "4. MAG IDLE" {
      }
      frame "5. PREP NEXT FIELD" {
        # "Prepares for next field by leaving persistenet mode"
        n69 = call "PREP FIELD.vi"("Numeric"=w358, "Lead- Mode Ramp Rate (A/s)"=w353, "PSU Status In"=w355, "MagQ in"=w356, "VISA Refnum in"=w354) -> ("error out"=w352:errorcluster, "Output (T)"=→"Output (T)":dbl, "MagQ out"=w357:refnum<queue>, "VISA Refnum out"=w351:refnum<visa-resource-name>)  [unwired: 3 in]
      }
      frame "6. APPLY NEXT FIELD" {
        # "Applies next field in index"
        n70 = call "APPLY FIELD.vi"("Numeric in"=w363, "error in (no error)"=w364, "PSU Status In"=w365, "MagQ in"=w360, "VISA Refnum in"=w366) -> ("error out"=w368:errorcluster, "PSU Status Out"=w361:T10, "MagQ out"=w369:refnum<queue>, "VISA Refnum out"=w362:refnum<visa-resource-name>, "Numeric out"=w359:i32)  [unwired: 2 in]
        n71 = Wait (ms)(milliseconds to wait=u32 5000) -> ()  [unwired: 1 out]
      }
      frame "7. PREP OFF" {
        # "Preps off by leaving P-mode"
        # "Assuming Heater is in off state to start."
        n72 = call <instrlib>:"Ramp.vi"("Error in (no error)"=w389, "Ramp Target"=T12."RAMP TO MID", "PSU Status In"=w390, "VISA Resource Name In"=w391) -> ("Error out"=w386:errorcluster, "PSU Status Out"=w387:T10, "VISA Resource Name Out"=w388:refnum<visa-resource-name>)  [unwired: 4 in, 1 out]
        n73 = call <instrlib>:"Get MID.vi"("Error in (no error)"=w386, "PSU Status In"=w387, "VISA Resource Name In"=w388) -> ("MID Setpoint (T)"=w379:dbl, "PSU Status Out"=w384:T10, "VISA Resource Name Out"=w385:refnum<visa-resource-name>)  [unwired: 3 in, 3 out]
        n74 = call <instrlib>:"Get Output.vi"("PSU Status In"=w384, "VISA Resource Name In"=w385) -> ("Error out"=w374:errorcluster, "PSU Status Out"=w375:T10, "VISA Resource Name Out"=w377:refnum<visa-resource-name>, "Output (T)"=w380:dbl)  [unwired: 4 in, 2 out]
        n75 = Subtract(x=w379, y=w380) -> (x-y=w383:dbl)
        n76 = Flush Queue(queue=w381) -> (queue out=w378:refnum<queue>)  [unwired: 1 in, 2 out]
        n77 = Less Or Equal?(x=w383, y=0.002) -> (x <= y?=w376:bool)
        n78 = call "MAG PREP.vi"("VISA In"=w377, "MagQ"=w378, "Boolean"=w376, "PSU Status In"=w375, "Error In"=w374) -> ("VISA Out"=w373:refnum<visa-resource-name>, "MagQ"=w372:refnum<queue>, "PSU Status Out"=w371:T10, "error out"=w370:errorcluster)  [unwired: 7 in]
      }
      frame "8. MAG OFF (Reset)" {
        # "Shutsdown magnet"
        n79 = call <instrlib>:"Get Output.vi"("Error in (no error)"=w406, "PSU Status In"=w405, "VISA Resource Name In"=w407) -> ("Error out"=w399:errorcluster, "PSU Status Out"=w401:T10, "VISA Resource Name Out"=w402:refnum<visa-resource-name>, "Output (T)"=w404:dbl)  [unwired: 3 in, 2 out]
        n80 = Less Or Equal?(x=w404, y=0.001) -> (x <= y?=w398:bool)
        n81 = call "MAG OFF.vi"("VISA Resource Name Out"=w402, "MagQ"=w400, "Boolean"=w398, "PSU Status Out"=w401, "Error out"=w399) -> ("VISA Resource Name Out 2"=w397:refnum<visa-resource-name>, "MagQ 2"=w395:refnum<queue>, "Boolean 2"=w394:bool, "PSU Status Out 2"=w396:T10, "error out"=w393:errorcluster)  [unwired: 6 in]
      }
    }
  }
  n82 = while {
    tunnel: w52 -> [w424]
    shift-right: [w408] -> _
    shift-left: _ -> [w422]
    tunnel: [w421] -> _
    tunnel: [w419] -> _
    tunnel: [w417] -> w45
    tunnel: w13 -> [w415]
    tunnel: w51 -> [w414]
    tunnel: "Field and Temp Range" -> [w413]
    tunnel: w5 -> [w412]
    tunnel: [w411] -> _
    tunnel: w8 -> [w410]
    tunnel: [w409] -> _
    stop <- w416 stop-if-true
    # "Sweep Handler"
    n83 = Dequeue Element(queue=w424, error in (no error)=w414) -> (queue out=w420:refnum<queue>, element=w423:T6, error out=w418:errorcluster)  [unwired: 1 in, 1 out]
    n84 = Unbundle By Name(w423) -> ("Sweep States"=w425:T4)
    n85 = case shown="\"SET TEMP & FIELD\"" w425 {
      tunnel: w422 -> [_ w437 _ w448 w458]
      tunnel: [_ w438 _ w443 w454] -> w421
      tunnel: w420 -> [w429 w436 _ w446 w459]
      tunnel: [_ w437 _ w447 w458] -> w408
      tunnel: [w427 w435 _ w444 w459] -> w419
      tunnel: w418 -> [_ w433 _ w439 w455]
      tunnel: [_ w431 _ w441 w452] -> w417
      tunnel: [_ _ _ _ w457] -> w416
      tunnel: w415 -> [_ w434 _ w445 w456]
      tunnel: w413 -> [_ _ _ _ _]
      tunnel: w412 -> [w428 _ _ _ w453]
      tunnel: [w426 _ _ _ w451] -> w411
      tunnel: w410 -> [_ w432 _ w442 w450]
      tunnel: [_ w430 _ w440 w449] -> w409
      frame "NO CHANGE" {
        # "If no change, will just scan/bias"
        n86 = call "No_Change.vi"("ScanQ in"=w428, "Queue in"=w429) -> ("ScanQ out"=w426:refnum<queue>, "Queue out"=w427:refnum<queue>)  [unwired: 8 in]
      }
      frame "SET TEMP & FIELD" {
        # "Inits Mag and TC"
        n87 = call "Set_Temp_Field.vi"("error in (no error)"=w433, "TempQ in"=w432, "MagQ in"=w434, "Queue in"=w436) -> ("error out"=w431:errorcluster, "TempQ out"=w430:refnum<queue>, "MagQ out"=w438:refnum<queue>, "Queue out"=w435:refnum<queue>)  [unwired: 4 in]
      }
      frame "SWEEP IDLE" {
      }
      frame "NEXT TEMP & FIELD" {
        # "Searches for next B and T"
        n88 = call "Next_Temp_Field.vi"("Numeric in"=w448, "error in (no error)"=w439, "TempQ in"=w442, "MagQ in"=w445, "Queue in"=w446) -> ("error out"=w441:errorcluster, "TempQ out"=w440:refnum<queue>, "MagQ out"=w443:refnum<queue>, "Queue out"=w444:refnum<queue>, "Numeric out"=w447:i32)  [unwired: 2 in]
      }
      frame "SWEEP DONE" {
        # "Shutsdown instruments"
        n89 = call "Shutdown.vi"("error in (no error)"=w455, "TempQ in"=w450, "ScanQ in"=w453, "Queue in"=w456) -> ("error out"=w452:errorcluster, "TempQ out"=w449:refnum<queue>, "ScanQ out"=w451:refnum<queue>, "Queue out"=w454:refnum<queue>, "Boolean"=w457:bool)  [unwired: 3 in]
      }
    }
    "Current Index" <- w408
  }
  n90 = while {
    tunnel: w14 -> [w463]
    tunnel: [w462] -> w46
    tunnel: w5 -> [w460]
    stop <- w461 stop-if-true
    # "Next Temp Trigger"
    n91 = event shown="[0] \"Start\": Value Change" {
      selector: _ -> [_ _]
      dyn-events: _ -> [_ _]
      timeout: _ -> [_ _]
      tunnel: w463 -> [_ w473]
      tunnel: [w468 w476] -> w462
      tunnel: [_ w474] -> w461
      tunnel: w460 -> [w466 _]
      event "Start": Value Change {
        n92 = event-data() -> ()  [unwired: 1 in, 6 out]
        n93 = Bundle By Name(cluster=T11 {"Setpoint (I)"=[], "Bias (V)"=[], "Number of scans"=1, "Port number (3364)"=3364, "Avoid zero threshold (V)"=0.004999999888241291, "Current State"=enum."1. BIAS"} ("element"), "Current State"=T5."1. BIAS") -> (w465:T11)
        n94 = Enqueue Element(queue=w466, element=w465) -> (error out=w468:errorcluster)  [unwired: 2 in, 2 out]
      }
      event "stop": Value Change {
        n95 = event-data() -> ()  [unwired: 1 in, 1 out]
        n96 = Bundle By Name(cluster=T6 {"Temps(K)"=[], "Fields(T)"=[], "Sweep States"=enum."SET TEMP & FIELD"} ("Temp and Field Range"), "Sweep States"=T4."SWEEP DONE") -> (w470:T6)
        n97 = Flush Queue(queue=w473) -> (queue out=w472:refnum<queue>)  [unwired: 1 in, 2 out]
        n98 = Enqueue Element At Opposite End(queue=w472, element=w470) -> (error out=w476:errorcluster)  [unwired: 2 in, 2 out]
        n99 = case shown="True" "stop" {
          tunnel: [FALSE ("stop 2") TRUE ("stop 2")] -> w474
          frame False {
          }
          frame True {
          }
        }
      }
    }
  }
  n100 = Release Queue(queue=w17, error in (no error)=w16) -> (error out=w10:errorcluster)  [unwired: 1 in, 2 out]
  n101 = Release Queue(queue=w56, error in (no error)=w55) -> (error out=w31:errorcluster)  [unwired: 1 in, 2 out]
  n102 = VISA Clear(VISA resource name=w32, error in (no error)=w31) -> (VISA resource name out=w30:refnum<visa-resource-name>, error out=w29:errorcluster)
  n103 = VISA Close(VISA resource name=w30, error in (no error)=w29) -> (error out=w54:errorcluster)
  n104 = Release Queue(queue=w36, error in (no error)=w35) -> (error out=w9:errorcluster)  [unwired: 1 in, 2 out]
  n105 = Build Array(w46, w45, w54, w10, w9) -> (→"Errors":errorcluster[])
